vi "TETRIX RC.vi"(8 "error in 2":errorcluster, 10 "RC":u16[](array[numeric])=[1500, 1500, 1500, 1500, 1500, 1500, 1500], 11 "KNR in 3":T1) -> (0 "error out 4":errorcluster caption="error out", 3 "KNR out 4":T1)   [LabVIEW 2013]
uses:
  <userlib>/KNR OS 3.0 LabVIEW Toolkit/Type Definition/KNR3 Reference.ctl
  <userlib>/_FPGA Interface Advanced Tools/FPGA Interface Base/FPGA Interface Base.lvclass
  <userlib>/KNR OS 3.0 LabVIEW Toolkit/Type Definition/Resource.ctl
  <userlib>/KNR OS 3.0 LabVIEW Toolkit/support SubVI/_Controls/Lego Port.ctl
panel:
  out "Servo In Position?":bool
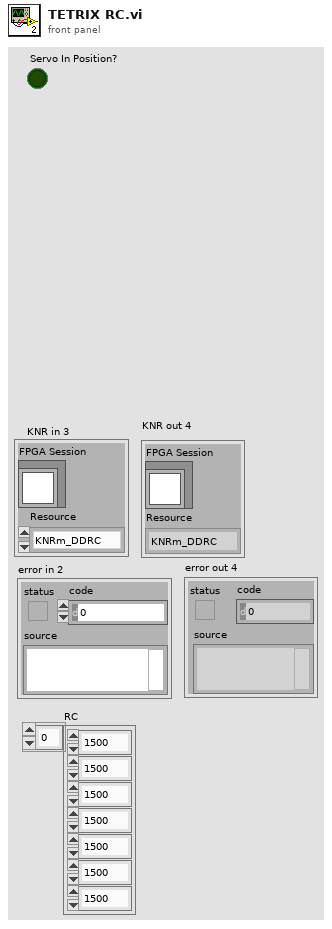
[diagram p1: front panel]
types:
  T1 = typedef "KNR3 Reference.ctl" = cluster{"FPGA Session":refnum<class "FPGA Interface Base.lvclass">, "Resource":T2}
  T2 = typedef "Resource.ctl" = enum16{"KNRm_DDRC", "KNRm_DDDD", "KNRm_DDDR", "KNRm_DDDC", "KNR"}
  T3 = typedef "Lego Port.ctl" = enum8{"L1", "LS1", "LS3", "LS4", "LS2"}
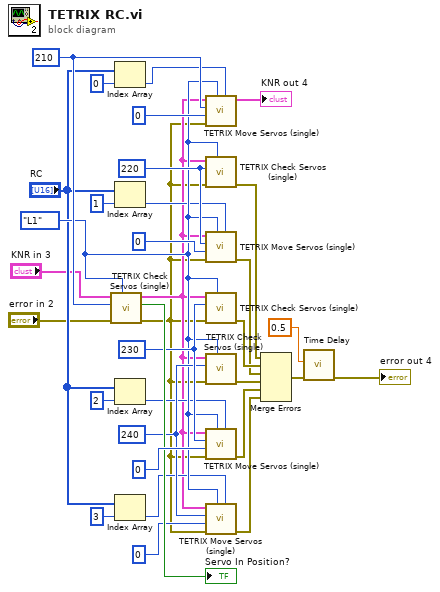
[diagram p0: block diagram]
diagram:
  w22 = u32 240 ("Servo ID(110)")
  w23 = u32 230 ("DC Motor ID(110)")
  w26 = u32 220 ("DC Motor ID(110)")
  w27 = u32 210 ("DC Motor ID(110)")
  w20 = Lego_Port."L1" ("Port (LS1)")
  n1 = call <userlib>:"TETRIX Check Servos (single).vi"("Port (LS1)"=w20, "error in"="error in 2", "Servo ID(110)"=w27, "KNR in"="KNR in 3") -> ("error out"=w11:errorcluster, "Servo In Position?"=→"Servo In Position?":bool, "KNR out"=w12:T1)  [unwired: 5 in]
  n2 = Index Array(array="RC", index=0) -> (element=w25:u16)
  n3 = Index Array(array="RC", index=1) -> (element=w15:u16)
  n4 = Index Array(array="RC", index=2) -> (element=w16:u16)
  n5 = Index Array(array="RC", index=3) -> (element=w19:u16)
  n6 = call <userlib>:"TETRIX Move Servos (single).vi"("Servo Position(0)"=w25, "Port (LS1)"=w20, "error in"=w11, "Update Interval (0)"=u8 0, "Servo ID(110)"=w27, "KNR in"=w12) -> ("KNR out"=→"KNR out 4":T1)  [unwired: 4 in, 1 out]
  n7 = call <userlib>:"TETRIX Check Servos (single).vi"("Port (LS1)"=w20, "error in"=w11, "Servo ID(110)"=w26, "KNR in"=w12) -> ("error out"=w9:errorcluster)  [unwired: 5 in, 2 out]
  n8 = call <userlib>:"TETRIX Move Servos (single).vi"("Servo Position(0)"=w15, "Port (LS1)"=w20, "error in"=w11, "Update Interval (0)"=u8 0, "Servo ID(110)"=w26, "KNR in"=w12) -> ("error out"=w7:errorcluster)  [unwired: 4 in, 1 out]
  n9 = call <userlib>:"TETRIX Check Servos (single).vi"("Port (LS1)"=w20, "error in"=w11, "Servo ID(110)"=w23, "KNR in"=w12) -> ("error out"=w8:errorcluster)  [unwired: 5 in, 2 out]
  n10 = call <userlib>:"TETRIX Check Servos (single).vi"("Port (LS1)"=w20, "error in"=w11, "Servo ID(110)"=w22, "KNR in"=w12) -> ("error out"=w6:errorcluster)  [unwired: 5 in, 2 out]
  n11 = call <userlib>:"TETRIX Move Servos (single).vi"("Servo Position(0)"=w16, "Port (LS1)"=w20, "error in"=w11, "Update Interval (0)"=u8 0, "Servo ID(110)"=w23, "KNR in"=w12) -> ("error out"=w5:errorcluster)  [unwired: 4 in, 1 out]
  n12 = call <userlib>:"TETRIX Move Servos (single).vi"("Servo Position(0)"=w19, "Port (LS1)"=w20, "error in"=w11, "Update Interval (0)"=u8 0, "Servo ID(110)"=w22, "KNR in"=w12) -> ("error out"=w4:errorcluster)  [unwired: 4 in, 1 out]
  n13 = Merge Errors(w9, w8, w7, w6, w5, w4) -> (w3:errorcluster)
  n14 = call "Time Delay"("error in (no error)"=w3, "Delay Time (s)"=0.5) -> ("error out"=→"error out 4":errorcluster)  [unwired: 9 in]
